vi "loadDataNode.vi"(8 "error in (no error)":errorcluster, 9 "CnfgEditorDir":path, 10 "XML Refnum in":refnum<file>, 11 "xceDataNode in":refnum<class "xceDataNode.lvclass">) -> (0 "error out":errorcluster, 2 "XML Refnum out":refnum<file>, 3 "xceDataNode out":refnum<class "xceDataNode.lvclass">)   [LabVIEW 2013, in "xceDataNode.lvclass"]
doc: "Loads a xceDataNode object from file, and then adds the link between this loaded node, and its supernode."
uses:
  xceDataNode.lvclass
  xceDataNode.lvclass/xceDataNode.ctl
  XML Parser/lineCounter_action.ctl
  xceNode/xceNode.lvclass
  XML Parser/XML Parser.lvclass
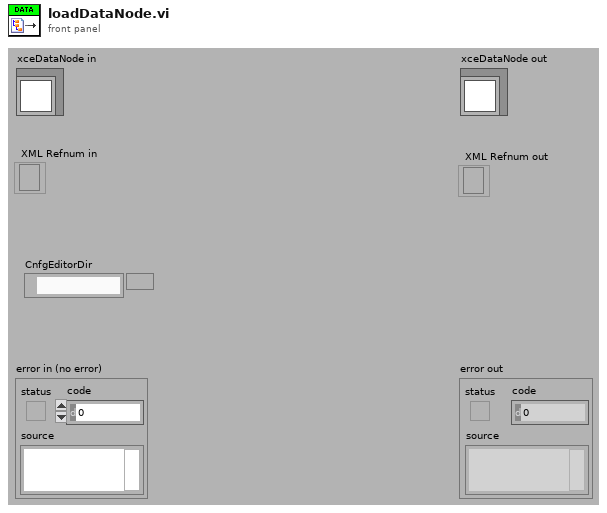
[diagram p1: front panel]
types:
  T1 = typedef "XML Parser.lvclass/lineCounter_action.ctl" = enum16{"Init", "Reset", "Increment", "Get Current Line"}
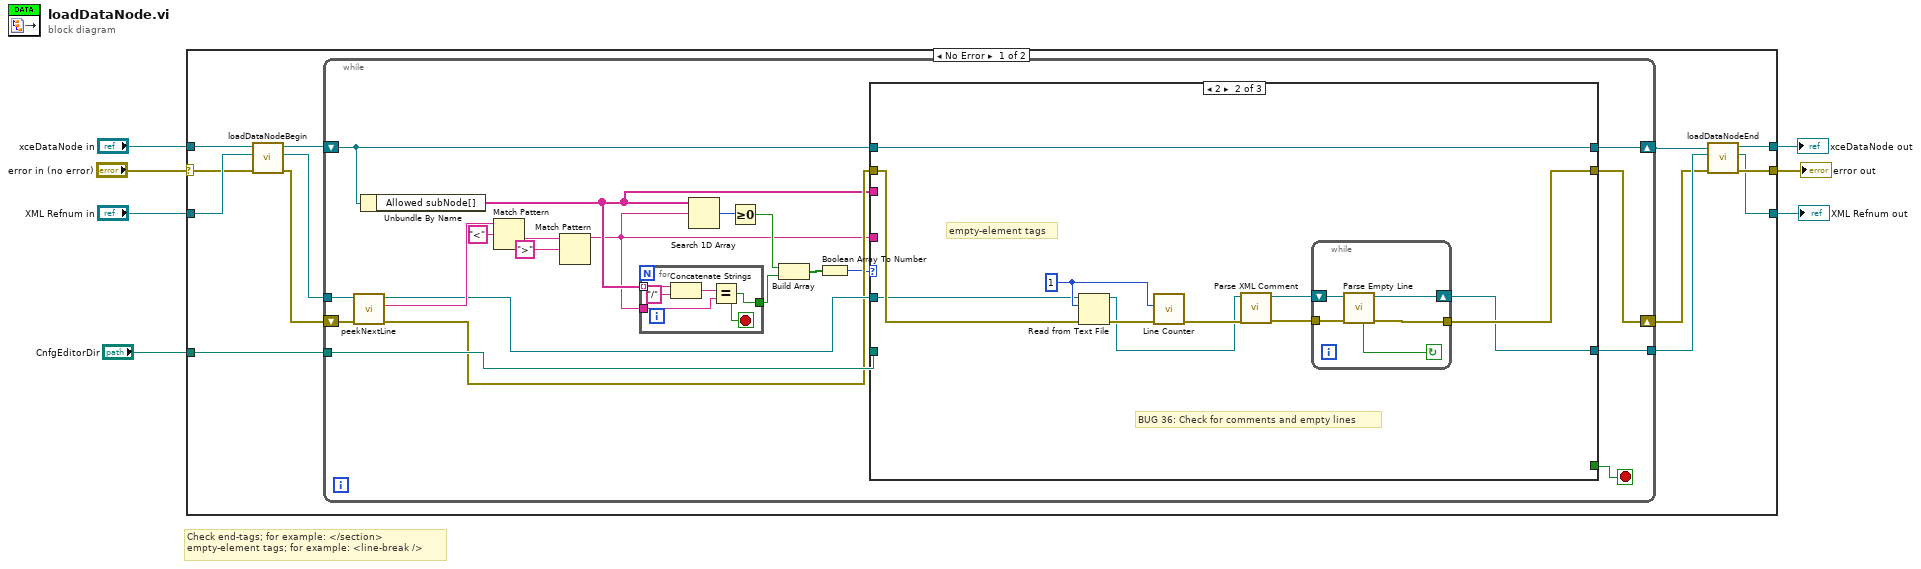
[diagram p0: block diagram]
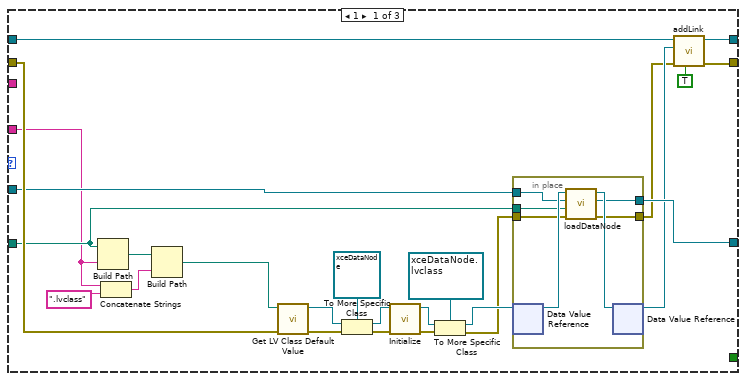
[diagram p2: hidden frame]
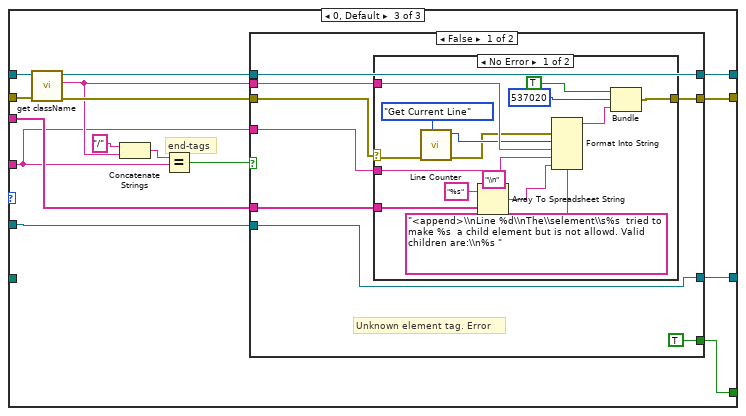
[diagram p3: hidden frame]
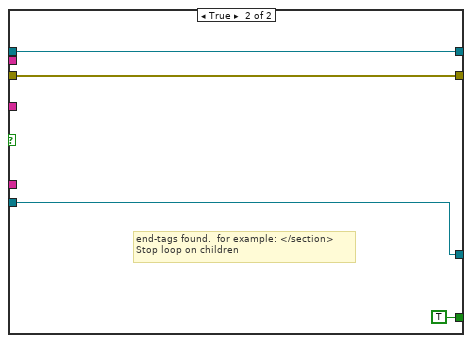
[diagram p5: hidden frame]
diagram:
  # "Check end-tags; for example: </section>\nempty-element tags; for example: <line-break />"
  n1 = case shown="No Error" "error in (no error)" {
    selector: "error in (no error)" -> [w11 w140]
    tunnel: [w14 w140] -> w6
    tunnel: [w17 w139] -> w4
    tunnel: "xceDataNode in" -> [w20 w139]
    tunnel: "XML Refnum in" -> [w19 w138]
    tunnel: [w13 w138] -> w2
    tunnel: "CnfgEditorDir" -> [w12 _]
    frame No Error {
      n2 = call-dynamic "loadDataNodeBegin.vi"("error in (no error)"=w11, "XML Refnum in"=w19, "xceDataNode in"=w20) -> ("error out"=w10:errorcluster, "XML Refnum out"=w18:refnum<file>, "xceDataNode out"=w8:refnum<class "xceDataNode.lvclass">)  [unwired: 6 in]
      n3 = while {
        tunnel: w18 -> [w41]
        tunnel: [w33] -> w16
        tunnel: w12 -> [w31]
        shift-right: [w29] -> w9
        shift-left: w8 -> [w30]
        shift-right: [w32] -> w15
        shift-left: w10 -> [w40]
        stop <- w35 stop-if-true
        n4 = call "peekNextLine.vi"("error in"=w40, "file* in"=w41) -> ("error out"=w28:errorcluster, "nextLine"=w39:string, "file* out"=w34:refnum<file>)  [unwired: 7 in]
        n5 = Unbundle By Name(w30) -> ("Allowed subNode[]"=w23:string[])
        n6 = Match Pattern(string=w39, regular expression="<") -> (after substring=w37:string)  [unwired: 1 in, 3 out]
        n7 = Match Pattern(string=w37, regular expression=">") -> (before substring=w22:string)  [unwired: 1 in, 3 out]
        n8 = for {
          tunnel: w23 -> [w46] mode=indexing
          tunnel: [w43] -> w21
          tunnel: w22 -> [w42]
          stop <- w43 stop-if-true
          n9 = Concatenate Strings(w46, "/" ("string")) -> (w44:string)
          n10 = Equal?(x=w44, y=w42) -> (x = y?=w43:bool)
        }
        n11 = Search 1D Array(1D array=w23, element=w22) -> (index of element=w27:i32)  [unwired: 1 in]
        n12 = Greater Or Equal To 0?(x=w27) -> (x >= 0?=w26:bool)
        n13 = Build Array(w26, w21) -> (w25:bool[])
        n14 = Boolean Array To Number(Boolean array=w25) -> (number=w24:u32)
        n15 = case shown="2" w24 {
          tunnel: [_ _ w98] -> w35
          tunnel: w34 -> [w56 w87 w97]
          tunnel: w28 -> [w64 w88 w108]
          tunnel: [w55 w79 w96] -> w33
          tunnel: [w49 w80 w104] -> w32
          tunnel: w22 -> [w47 _ w99]
          tunnel: w31 -> [w58 _ _]
          tunnel: w30 -> [w53 w85 w109]
          tunnel: [w52 w85 w105] -> w29
          tunnel: w23 -> [_ _ w103]
          frame 1 {
            n16 = Build Path(base path=w58, name or relative path=w47) -> (appended path=w57:path)
            n17 = Concatenate Strings(w47, ".lvclass" ("string")) -> (w66:string)
            n18 = Build Path(base path=w57, name or relative path=w66) -> (appended path=w67:path)
            n19 = call <vilib>:"Get LV Class Default Value.vi"("error in (no error)"=w64, "class path"=w67) -> ("error out"=w70:errorcluster, "object"=w68:refnum<class>)  [unwired: 8 in]
            n20 = To More Specific Class(target class=refnum<class "xceDataNode.lvclass"> refnum ("xceDataNode.lvclass"), reference=w68, error in=w70) -> (specific class reference=w69:refnum<class "xceDataNode.lvclass">, error out=w71:errorcluster)
            n21 = call-dynamic "Initialize.vi"("error in"=w71, "xceDataNode in"=w69) -> ("error out"=w63:errorcluster, "Node*"=w62:refnum<data-value>)  [unwired: 8 in]
            n22 = To More Specific Class(target class=refnum<data-value> refnum ("data value reference"), reference=w62, error in=w63) -> (specific class reference=w59:refnum<data-value>, error out=w54:errorcluster)
            n23 = in-place {
              in-place-border: w58 -> [w77]
              in-place-border: w56 -> [w76]
              in-place-border: [w74] -> w55
              in-place-border: w54 -> [w73]
              in-place-border: [w72] -> w50
              n24 = in-place-dvr #1(w59) -> (w78:refnum<class "xceDataNode.lvclass">)  [unwired: 1 out]
              n25 = call "loadDataNode.vi"("error in (no error)"=w73, "CnfgEditorDir"=w77, "XML Refnum in"=w76, "xceDataNode in"=w78) -> ("error out"=w72:errorcluster, "XML Refnum out"=w74:refnum<file>, "xceDataNode out"=w75:refnum<class "xceDataNode.lvclass">)  [unwired: 5 in]
              n26 = in-place-dvr #1(w75) -> (w51:refnum<data-value>)  [unwired: 1 out]
            }
            n27 = call "addLink.vi"("Append to End"=TRUE, "error in (no error)"=w50, "subNode in"=w51, "superNode in"=w53) -> ("error out"=w49:errorcluster, "superNode out"=w52:refnum<class "xceDataNode.lvclass">)  [unwired: 5 in, 1 out]
          }
          frame 2 {
            w89 = 1 ("count")
            # "BUG 36: Check for comments and empty lines"
            # "empty-element tags"
            n28 = Read from Text File(file (use dialog)=w87, count=w89, error in=w88) -> (refnum out=w83:refnum<file>, error out=w86:errorcluster)  [unwired: 1 in, 2 out]
            n29 = call "Line Counter.vi"("error in (no error)"=w86, "# of lines to increment (1)"=w89) -> ("error out"=w84:errorcluster)  [unwired: 8 in, 1 out]
            n30 = call "Parse XML Comment.vi"("error in (no error)"=w84, "XML Refnum in"=w83) -> ("error out"=w81:errorcluster, "XML Refnum out"=w82:refnum<file>)  [unwired: 6 in, 2 out]
            n31 = while {
              tunnel: w81 -> [w93]
              tunnel: [w91] -> w80
              shift-right: [w90] -> w79
              shift-left: w82 -> [w94]
              stop <- w92 continue-if-true
              n32 = call "Parse Empty Line.vi"("error in (no error)"=w93, "XML Refnum in"=w94) -> ("error out"=w91:errorcluster, "XML Refnum out"=w90:refnum<file>, "Empty Line Found"=w92:bool)  [unwired: 7 in]
            }
          }
          frame 0, Default {
            # "end-tags"
            n33 = call "get className.vi"("error in (no error)"=w108, "xceNode in"=w109) -> ("error out"=w107:errorcluster, "Class name"=w100:string, "xceNode out"=w106:refnum<class "xceDataNode.lvclass">)  [unwired: 7 in]
            n34 = Concatenate Strings("/" ("string"), w100) -> (w102:string)
            n35 = Equal?(x=w102, y=w99) -> (x = y?=w95:bool)
            n36 = case shown="False" w95 {
              tunnel: w100 -> [w115 _]
              tunnel: w99 -> [w114 _]
              tunnel: w107 -> [w110 w136]
              tunnel: w106 -> [w117 w137]
              tunnel: [w117 w137] -> w105
              tunnel: [w116 w136] -> w104
              tunnel: w103 -> [w113 _]
              tunnel: [TRUE TRUE] -> w98
              tunnel: w97 -> [w111 w134]
              tunnel: [w111 w134] -> w96
              frame False {
                # "Unknown element tag. Error"
                n37 = case shown="No Error" w110 {
                  selector: w110 -> [w118 w133]
                  tunnel: [w132 w133] -> w116
                  tunnel: w115 -> [w131 _]
                  tunnel: w114 -> [w130 _]
                  tunnel: w113 -> [w129 _]
                  frame No Error {
                    n38 = call "Line Counter.vi"("Action (Increment)"=lineCounter_action."Get Current Line", "error in (no error)"=w118) -> ("error out"=w122:errorcluster, "Current Line"=w123:i32)  [unwired: 8 in]
                    n39 = Array To Spreadsheet String(delimiter (Tab)="\\n", array=w129, 3:"%s" ("format string")) -> (spreadsheet string=w120:string)
                    n40 = Format Into String(format string="<append>\\nLine %d\\nThe\\selement\\s%s  tried to make %s  a child element but is not allowd. Valid children are:\\n%s ", error in=w122, w123, w131, w130, w120) -> (resulting string=w125:string)  [unwired: 1 in, 1 out]
                    n41 = Bundle("status"=TRUE, "code"=537020, w125) -> (w132:cluster{"status":bool, "code":i32, string})  [unwired: 1 out]
                  }
                  frame Error {
                  }
                }
              }
              frame True {
                # "end-tags found.  for example: </section>\nStop loop on children"
              }
            }
          }
        }
      }
      n42 = call-dynamic "loadDataNodeEnd.vi"("error in (no error)"=w15, "XML Refnum in"=w16, "xceDataNode in"=w9) -> ("error out"=w14:errorcluster, "XML Refnum out"=w13:refnum<file>, "xceDataNode out"=w17:refnum<class "xceDataNode.lvclass">)  [unwired: 6 in]
    }
    frame Error {
    }
  }
  "error out" <- w6
  "xceDataNode out" <- w4
  "XML Refnum out" <- w2
